vi "KVMap-Filter.vi"(8 "T->First/F->Second(F)":bool, 10 "filter":string, 11 "Cluster in":cluster{string[], string[]}) -> (3 "Cluster out":cluster{string[], string[]})   [LabVIEW 2017]
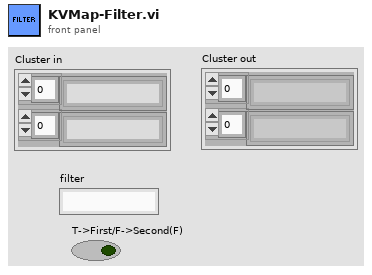
[diagram p1: front panel]
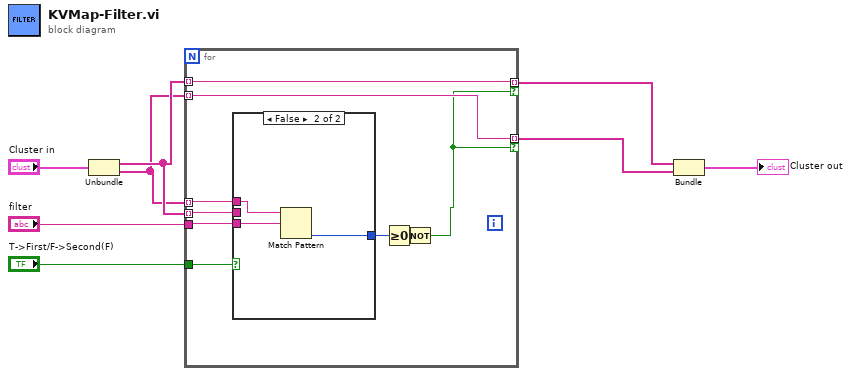
[diagram p0: block diagram]
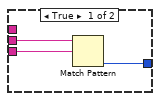
[diagram p2: hidden frame]
diagram:
  n1 = Unbundle("Cluster in") -> (w4:string[], w3:string[])
  n2 = for {
    tunnel: w3 -> [w17] mode=indexing
    tunnel: "T->First/F->Second(F)" -> [w16]
    tunnel: w4 -> [w15] mode=indexing
    tunnel: "filter" -> [w14]
    tunnel: [w11] -> w1 mode=indexing if=w9
    tunnel: w4 -> [w11] mode=indexing
    tunnel: [w10] -> w2 mode=indexing if=w9
    tunnel: w3 -> [w10] mode=indexing
    n3 = case shown="False" w16 {
      tunnel: w14 -> [w20 w23]
      tunnel: w15 -> [w19 _]
      tunnel: w17 -> [_ w22]
      tunnel: [w18 w21] -> w13
      frame True {
        n4 = Match Pattern(string=w19, regular expression=w20) -> (offset past match=w18:i32)  [unwired: 1 in, 3 out]
      }
      frame False {
        n5 = Match Pattern(string=w22, regular expression=w23) -> (offset past match=w21:i32)  [unwired: 1 in, 3 out]
      }
    }
    n6 = Greater Or Equal To 0?(x=w13) -> (x >= 0?=w12:bool)
    n7 = Not(x=w12) -> (.not. x?=w9:bool)
  }
  n8 = Bundle(w1, w2) -> (→"Cluster out":cluster{string[], string[]})  [unwired: 1 in]
